vi "Read single CAN.vi"(6 "timeout in ms (-1)":i32=-1, 8 "error in":errorcluster, 10 "ID":i32, 11 "CAN Session In":T2=refnum) -> (0 "error out":errorcluster, 2 "CAN Frame Out":T1 {"Data" format="%.0x"; "DataLength" format="%.0x"; "InfoB" format="%.0x"; "InfoA" format="%.0x"; "Type" format="%.0x"; "Identifier" format="%.0x"; "Timestamp" format="%.0x"}, 3 "CAN Session Out":T2)   [LabVIEW 2016]
doc: "The VI read a CAN packet (frame) from the CAN bus."
uses:
  Program Files (x86)/National Instruments/LabVIEW 2016/examples/robotics/EPOS2 CANOpen Driver/Low Level VIs/Typedefs/CAN Refnum.ctl
  Program Files (x86)/National Instruments/LabVIEW 2016/examples/robotics/EPOS2 CANOpen Driver/Low Level VIs/Typedefs/CAN Session Pointer.ctl
  Program Files (x86)/National Instruments/LabVIEW 2016/examples/robotics/EPOS2 CANOpen Driver/Low Level VIs/Typedefs/CAN Communication References.ctl
  Program Files (x86)/National Instruments/LabVIEW 2016/examples/robotics/EPOS2 CANOpen Driver/Low Level VIs/Typedefs/kill process notifier array.ctl
  Program Files (x86)/National Instruments/LabVIEW 2016/examples/robotics/EPOS2 CANOpen Driver/Low Level VIs/Typedefs/Write Queue.ctl
  Program Files (x86)/National Instruments/LabVIEW 2016/examples/robotics/EPOS2 CANOpen Driver/Low Level VIs/Typedefs/FPGA CAN Frame Cluster.ctl
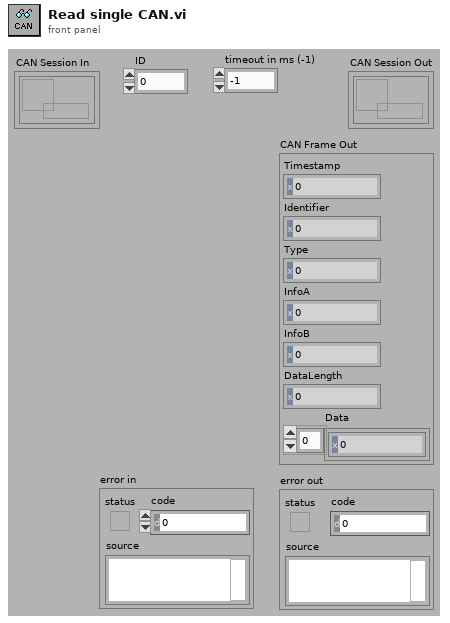
[diagram p1: front panel]
types:
  T1 = typedef "FPGA CAN Frame Cluster.ctl" = cluster{"Timestamp":u64, "Identifier":u32, "Type":u8, "InfoA":u8, "InfoB":u8, "DataLength":u8, "Data":u8[]}
  T2 = typedef "CAN Refnum.ctl" = refnum<k1>
  T3 = typedef "Write Queue.ctl" = refnum<queue>
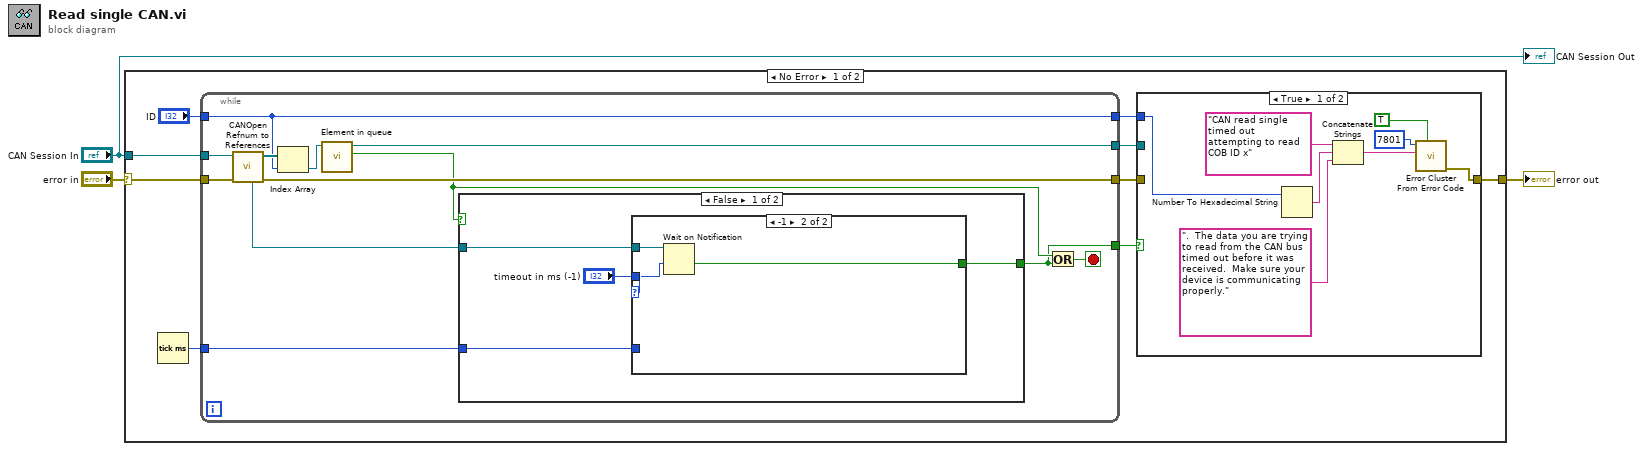
[diagram p0: block diagram]
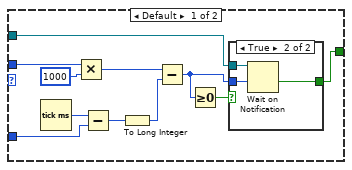
[diagram p2: hidden frame]
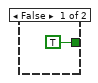
[diagram p3: hidden frame]
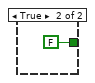
[diagram p4: hidden frame]
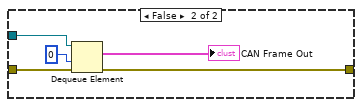
[diagram p5: hidden frame]
diagram:
  n1 = case shown="No Error" "error in" {
    selector: "error in" -> [w6 w61]
    tunnel: [w12 w61] -> w3
    tunnel: "CAN Session In" -> [w11 _]
    frame No Error {
      n2 = Tick Count (ms)() -> (millisecond timer value=w4:u32)
      n3 = while {
        tunnel: "ID" -> [w17]
        tunnel: w11 -> [w22]
        tunnel: [w17] -> w8
        tunnel: [w21] -> w9
        tunnel: [w20] -> w10
        tunnel: w6 -> [w19]
        tunnel: [w14] -> w5
        tunnel: w4 -> [w13]
        stop <- w18 stop-if-true
        n4 = call "CANOpen Refnum to References.vi"("error in (no error)"=w19, "CAN Session In"=w22) -> ("error out"=w20:errorcluster, "Read Queue Array"=w23:T3[], "New Frame Notifier"=w24:refnum<notifier>)  [unwired: 7 out]
        n5 = Index Array(array=w23, index=w17) -> (element=w16:T3)
        n6 = call "Element in queue.vi"("queue"=w16) -> ("Ready to read"=w15:bool, "queue out"=w21:T3)  [unwired: 9 in]
        n7 = case shown="False" w15 {
          tunnel: w24 -> [w28 _]
          tunnel: [w25 FALSE ("timed out?")] -> w14
          tunnel: w13 -> [w26 _]
          frame False {
            n8 = case shown="-1" "timeout in ms (-1)" {
              tunnel: w28 -> [w36 w46]
              tunnel: "timeout in ms (-1)" -> [w33 w45]
              tunnel: w26 -> [w32 _]
              tunnel: [w29 w44] -> w25
              frame Default {
                n9 = Tick Count (ms)() -> (millisecond timer value=w37:u32)
                n10 = Multiply(x=w33, y=1000) -> (x*y=w31:i32)
                n11 = Subtract(x=w37, y=w32) -> (x-y=w38:u32)
                n12 = To Long Integer(number=w38) -> (32bit integer=w39:i32)
                n13 = Subtract(x=w31, y=w39) -> (x-y=w30:i32)
                n14 = Greater Or Equal To 0?(x=w30) -> (x >= 0?=w35:bool)
                n15 = case shown="True" w35 {
                  tunnel: w36 -> [_ w43]
                  tunnel: [TRUE ("timed out?") w42] -> w29
                  tunnel: w30 -> [_ w41]
                  frame False {
                  }
                  frame True {
                    n16 = Wait on Notification(notifier=w43, timeout in ms (-1)=w41) -> (timed out?=w42:bool)  [unwired: 2 in, 3 out]
                  }
                }
              }
              frame -1 {
                n17 = Wait on Notification(notifier=w46, timeout in ms (-1)=w45) -> (timed out?=w44:bool)  [unwired: 2 in, 3 out]
              }
            }
          }
          frame True {
          }
        }
        n18 = Or(x=w15, y=w14) -> (x .or. y?=w18:bool)
      }
      n19 = case shown="True" w5 {
        tunnel: [w51 w58] -> w12
        tunnel: w10 -> [_ w57]
        tunnel: w9 -> [_ w59]
        tunnel: w8 -> [w48 _]
        frame True {
          n20 = Number To Hexadecimal String(2:w48) -> (0:w49:string)  [unwired: 1 in]
          n21 = Concatenate Strings("CAN read single timed out attempting to read COB ID x", w49, ".  The data you are trying to read from the CAN bus timed out before it was received.  Make sure your device is communicating properly.") -> (w53:string)
          n22 = call <vilib>:"Error Cluster From Error Code.vi"("show call chain? (False)"=TRUE, "error message (\"\")"=w53, "error code (0)"=7801) -> ("error out"=w51:errorcluster)  [unwired: 1 in, 5 out]
        }
        frame False {
          n23 = Dequeue Element(queue=w59, timeout in ms (-1)=0, error in (no error)=w57) -> (element=→"CAN Frame Out":T1, error out=w58:errorcluster)  [unwired: 2 out]
        }
      }
    }
    frame Error {
    }
  }
  "error out" <- w3
  "CAN Session Out" <- "CAN Session In"
